vi "BuildTestFromProjectItem_LibraryWithMember_BuildsTestSuiteWithTest.vi"() -> ()   [LabVIEW 2019, in "LVUnitTestBuilderTest.lvlib"]
uses:
  LVUnitTestBuilderTest.lvlib
  LVUnitTestBuilder/LVUnitTestBuilder.lvclass
  TestSuite/TestSuite.lvclass
  a12a2084-e44a-4edc-a973-f21fdd0e5ac6.vi
  Constraint/IsEqual/Create.vi
  Constraint/IsEqual/IsEqual.lvclass
panel:
  out "error out":errorcluster
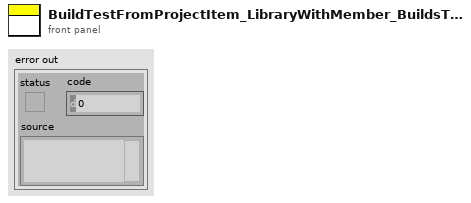
[diagram p1: front panel]
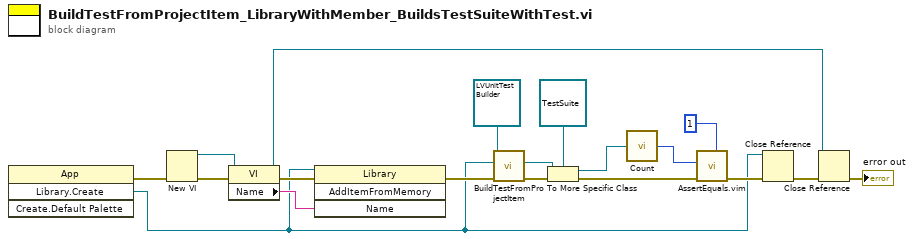
[diagram p0: block diagram]
diagram:
  n1 = invoke class="App" method="Library.Create"() -> (error out=w6:errorcluster, "Create Library"=w3:refnum<vi>)  [unwired: 4 in, 2 out]
  n2 = New VI(8:w6) -> (0:w9:errorcluster, 3:w8:refnum<vi>)  [unwired: 6 in]
  n3 = property class="VI"(reference=w8, error in=w9) -> (reference out=w1:refnum<vi>, error out=w5:errorcluster, "Name"=w7:string)
  n4 = invoke class="Library" method="AddItemFromMemory"(reference=w3, error in=w5, "Name"=w7) -> (error out=w4:errorcluster)  [unwired: 1 in, 3 out]
  n5 = call-dynamic "BuildTestFromProjectItem.vi"("error in (no error)"=w4, "ProjectItem Refnum"=w3, "LVUnitTestBuilder in"=refnum<class "LVUnitTestBuilder.lvclass"> refnum ("LVUnitTestBuilder")) -> ("error out"=w14:errorcluster, "Test"=w18:refnum<class "Test.lvclass">)  [unwired: 6 in, 1 out]
  n6 = To More Specific Class(target class=refnum<class "TestSuite.lvclass"> refnum ("TestSuite.lvclass"), reference=w18, error in=w14) -> (specific class reference=w16:refnum<class "TestSuite.lvclass">, error out=w13:errorcluster)
  n7 = call "Count.vi"("TestSuite In"=w16) -> ("Count"=w11:i32)
  n8 = call "AssertEquals.vim"("Expected"=1 ("Count"), "error in (no error)"=w13, "Actual"=w11) -> ("error out"=w12:errorcluster)  [unwired: 8 in]
  n9 = Close Reference(reference=w3, error in (no error)=w12) -> (error out=w15:errorcluster)
  n10 = Close Reference(reference=w1, error in (no error)=w15) -> (error out=→"error out":errorcluster)
